vi "GUI_HTT_MultiCamDriveExpAndComp.vi"() -> ()   [LabVIEW 2020]
uses:
  Shared/GUI_Template/GUI_master/tcp_new_data_event.ctl
  Shared/GUI_Template/GUI_master/tcp new data cluster.ctl
  General GUIs/Device GUIs/GUI_Cameras/Controls/Crosshair type def.ctl
  <userlib>/_OpenG.lib/array/array.llb/Filter 1D Array with Scalar (String)__ogtk.vi
panel:
  out "image1 4":T1(plugin-control)
  out "image1 3":T1(plugin-control)
  out "image1 2":T1(plugin-control)
  out "image::5":T1(plugin-control) caption="HTT-MagCam-04"
  out "image::4":T1(plugin-control) caption="HTT-MagCam-04"
  out "image::3":T1(plugin-control) caption="HTT-MagCam-04"
  out "image::2":T1(plugin-control) caption="HTT-MagCam-04"
  out "image1":T1(plugin-control)
  out "String 4":string="x1\ny1\nx2\ny2"
  out "String 3":string="x1\ny1\nx2\ny2"
  out "String 2":string="x1\ny1\nx2\ny2"
  out "String":string="x1\ny1\nx2\ny2"
  in  "visibility":bool=TRUE
  out "appended array":string[](array[string]) caption="XH"
  out "appended array 6":string[](array[string]) caption="XH"
  out "appended array 8":string[](array[string]) caption="XH"
  out "appended array 4":string[](array[string]) caption="XH"
  in  "UDP error message":string
  out "tcp data event 2":T2
  out "error IO 2":errorcluster
  in  "Color Box":u32(colorbox)
  in  "TargetSize.Y::5":dbl=45.0 caption="y" min=2.0 max=3000.0 format="%#_6f"
  in  "TargetSize.X::5":dbl=47.0 caption="x" min=2.0 max=3000.0 format="%#_6f"
  in  "TargetSize.Y::4":dbl=45.0 caption="y" min=2.0 max=3000.0 format="%#_6f"
  in  "TargetSize.X::4":dbl=47.0 caption="x" min=2.0 max=3000.0 format="%#_6f"
  in  "TargetSize.Y::3":dbl=163.0 caption="y" min=2.0 max=3000.0 format="%#_6f"
  in  "TargetSize.X::3":dbl=152.0 caption="x" min=2.0 max=3000.0 format="%#_6f"
  in  "TargetSize.Y::2":dbl=74.0 caption="y" min=2.0 max=3000.0 format="%#_6f"
  in  "TargetSize.X::2":dbl=75.0 caption="x" min=2.0 max=3000.0 format="%#_6f"
  in  "active cams":string
  out "CCDs":string[](array[string])
  out "Cameras":T3
  in  "Target.Y::5":dbl=45.0 caption="y" min=0.0 max=2000.0 format="%#_6f"
  in  "Target.X::5":dbl=47.0 caption="x" min=0.0 max=2000.0 format="%#_6f"
  in  "Target.Y::4":dbl=45.0 caption="y" min=0.0 max=2000.0 format="%#_6f"
  in  "Target.X::4":dbl=47.0 caption="x" min=0.0 max=2000.0 format="%#_6f"
  in  "Target.Y::3":dbl=163.0 caption="y" min=0.0 max=2000.0 format="%#_6f"
  in  "Target.X::3":dbl=152.0 caption="x" min=0.0 max=2000.0 format="%#_6f"
  in  "Target.Y::2":dbl=74.0 caption="y" min=0.0 max=2000.0 format="%#_6f"
  in  "Target.X::2":dbl=75.0 caption="x" min=0.0 max=2000.0 format="%#_6f"
  out "error out":errorcluster
  in  "triggerdelay::5":dbl=0.001 caption="triggerdelay" min=0.0 max=1000000.0 format="%_4p"
  in  "triggerdelay::4":dbl=0.001 caption="triggerdelay" min=0.0 max=10000000.0 format="%_4p"
  in  "triggerdelay::3":dbl=0.001 caption="triggerdelay" min=0.0 max=1000000.0 format="%_4p"
  in  "triggerdelay::2":dbl=0.001 caption="triggerdelay" min=0.0 max=1000000.0 format="%_4p"
  in  "trigger::5":bool caption="Trigger"
  in  "centroidy::5":dbl=0.001 caption="centroid y" min=0.0 max=0.0 format="%_4f"
  in  "centroidx::5":dbl=0.001 caption="centroid x" min=0.0 max=0.0 format="%_4f"
  in  "exposure::5":dbl=0.001 caption="exposure" min=1.0 max=10000000.0 format="%_4p"
  in  "GUIdevice 5":string="BellaCam25_2_cpoint2"
  in  "trigger::4":bool caption="Trigger"
  in  "centroidy::4":dbl=0.001 caption="centroid y" min=0.0 max=0.0 format="%_4f"
  in  "centroidx::4":dbl=0.001 caption="centroid x" min=0.0 max=0.0 format="%_4f"
  in  "exposure::4":dbl=0.001 caption="exposure" min=0.0001 max=1.0 format="%_4p"
  in  "GUIdevice 4":string="BellaCam13_1_cpoint1"
  in  "trigger::3":bool caption="Trigger"
  in  "centroidy::3":dbl=0.001 caption="centroid y" min=0.0 max=0.0 format="%_4f"
  in  "centroidx::3":dbl=0.001 caption="centroid x" min=0.0 max=0.0 format="%_4f"
  in  "exposure::3":dbl=0.001 caption="exposure" min=1e-05 max=1.0 format="%_4p"
  in  "GUIdevice 3":string="BellaCam13_3_tpoint2"
  in  "trigger::2":bool caption="Trigger"
  in  "centroidy::2":dbl=0.001 caption="centroid y" min=0.0 max=0.0 format="%_4f"
  in  "centroidx::2":dbl=0.001 caption="centroid x" min=0.0 max=0.0 format="%_4f"
  in  "exposure::2":dbl=0.001 caption="exposure" min=1.0 max=10000000.0 format="%_4p"
  in  "GUIdevice 2":string="BellaCam25_1_tpoint1"
  out "tcp data event":T2
  in  "Refresh Button":bool caption="Update Crosshairs"
  in  "Select device":string(combo)="FrogHPD"
  in  "stop":bool
  in  "GUIdevice 1":string="HPD_CCD"
  # "XHair location"
  # "XHair location"
  # "XHair size"
  # "XHair size"
  # "XHair location"
  # "XHair size"
  # "XHair size"
  # "XHair location"
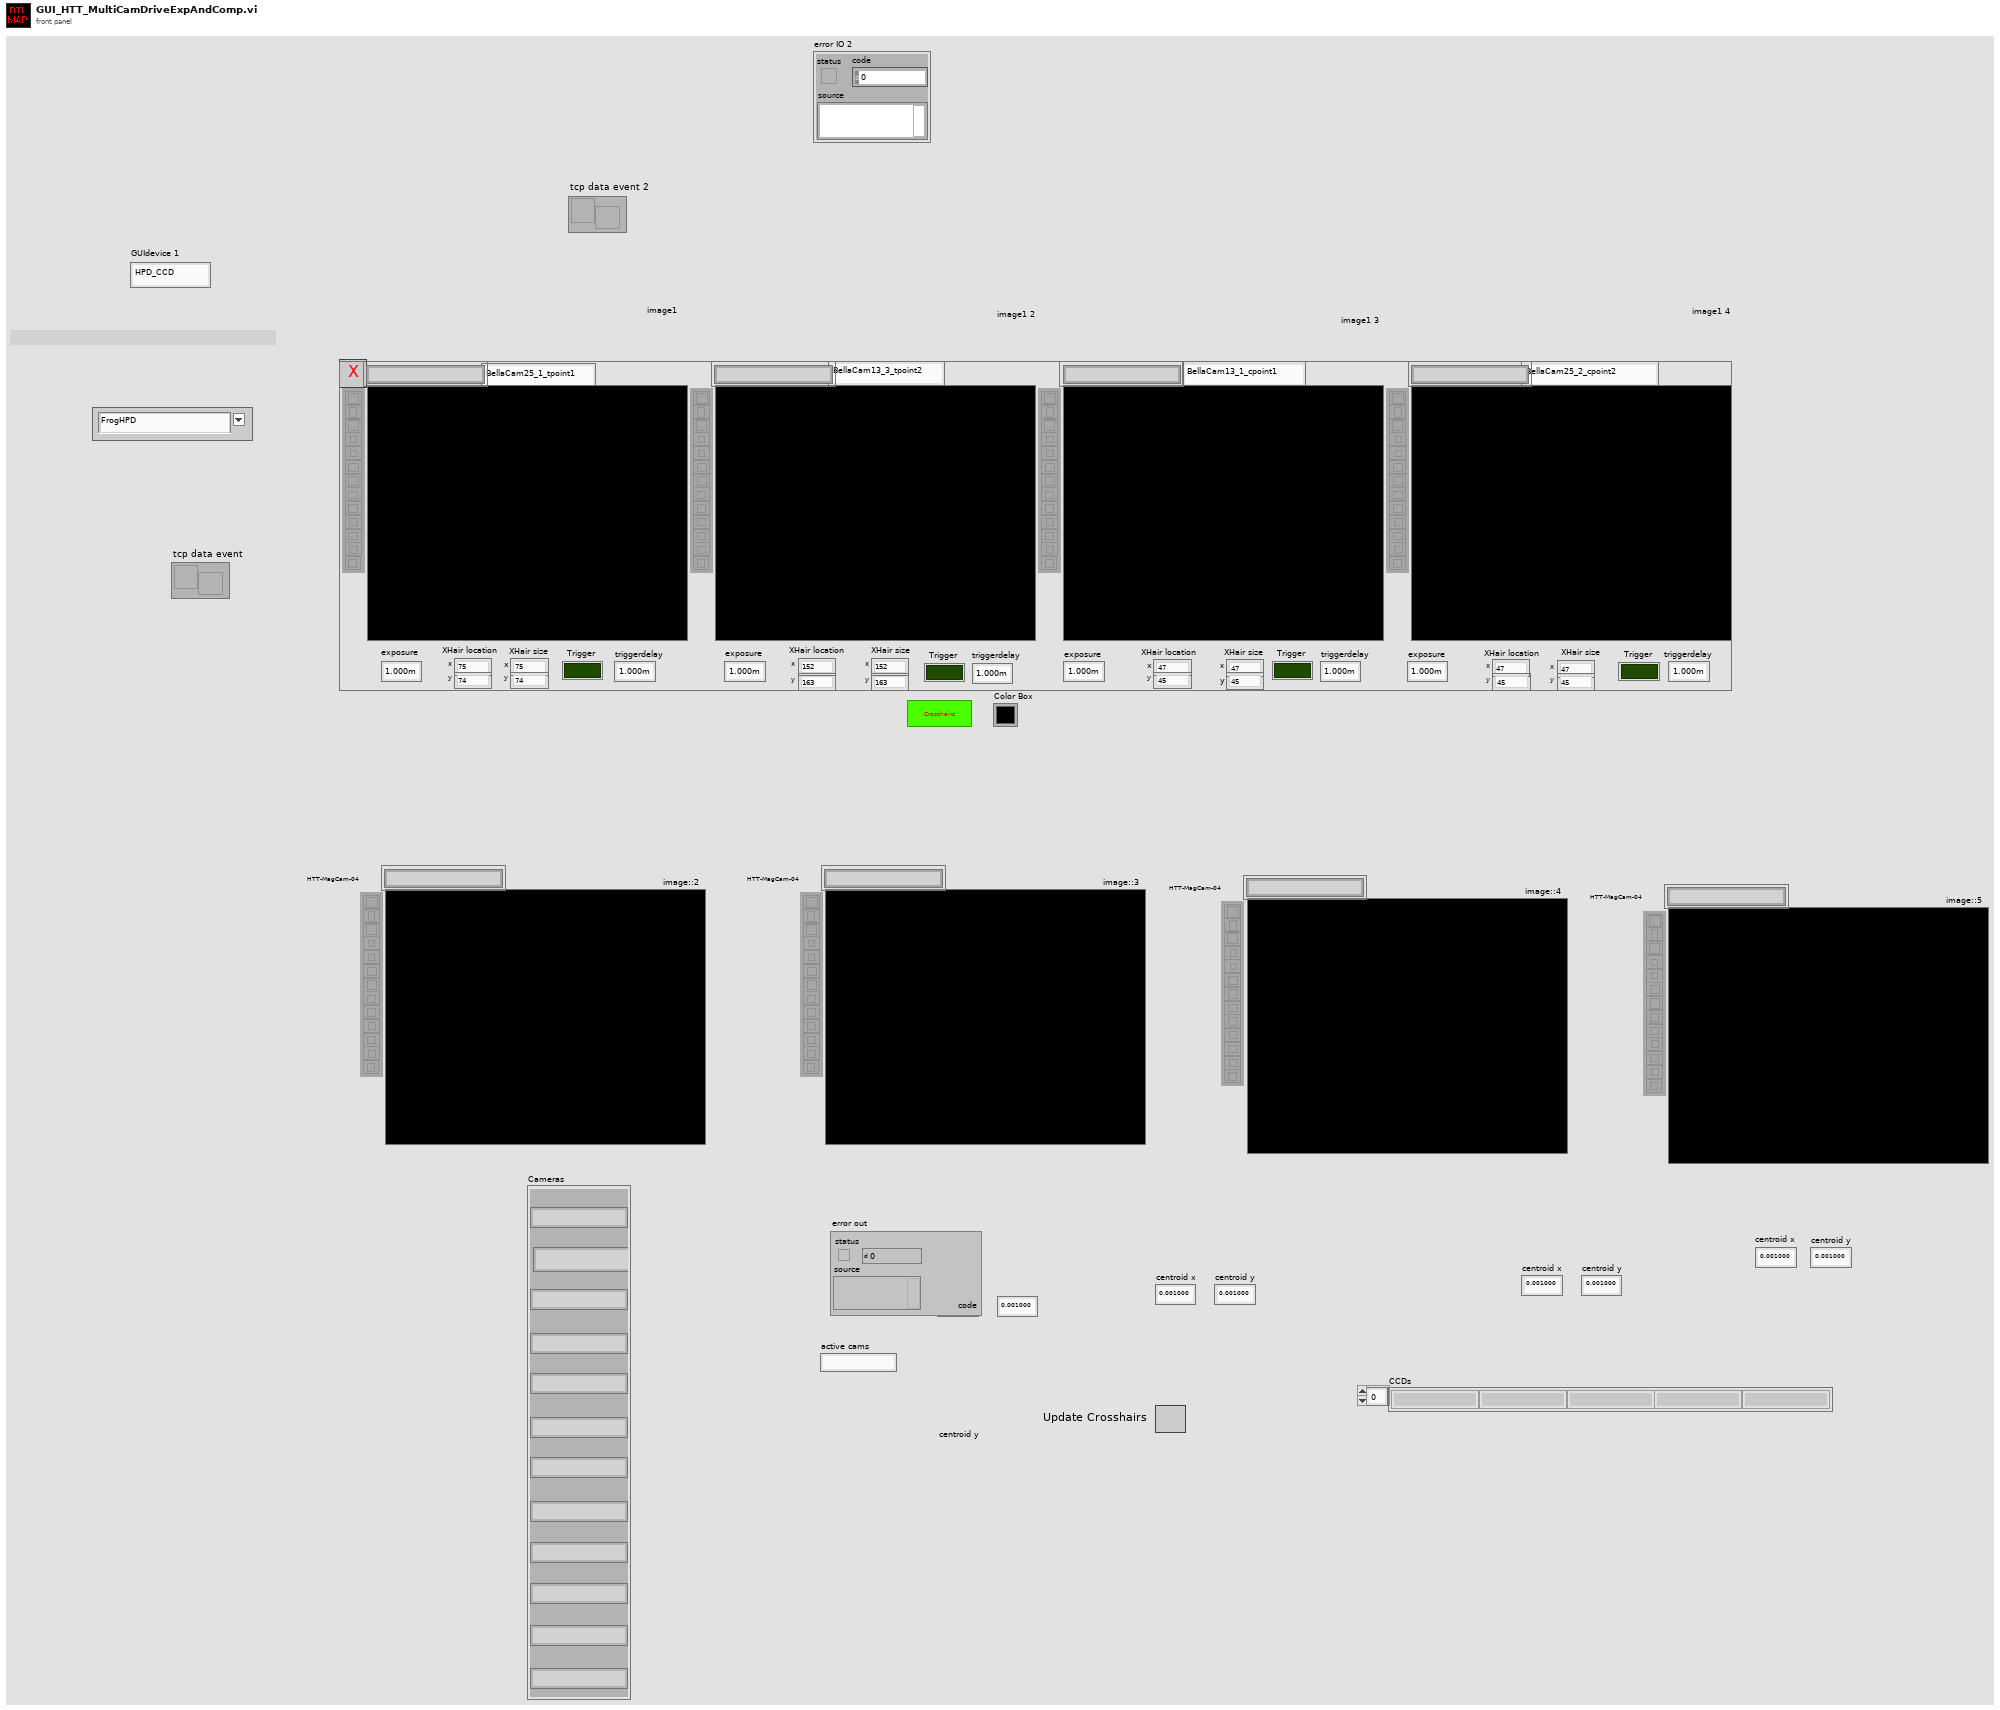
[diagram p1: front panel]
types:
  T1 = typedef "IMAQ Image.ctl" = refnum<image>
  T2 = typedef "tcp_new_data_event.ctl" = refnum<user-event>
  T3 = cluster{"[0]":string, "[1]":string, "[2]":string, "[3]":string, "[4]":string, "[5]":string, "[6]":string, "[7]":string, "[8]":string, "[8] 2":string, "[8] 3":string, "[8] 4":string}
  T4 = typedef "Image Type" = u32
  T5 = cluster{"Target.X::2":refnum<vi>, "Target.Y::2":refnum<vi>}
  T6 = cluster{"Target.X::3":refnum<vi>, "Target.Y::3":refnum<vi>}
  T7 = cluster{"Target.X::4":refnum<vi>, "Target.Y::4":refnum<vi>}
  T8 = cluster{"Target.X::5":refnum<vi>, "Target.Y::5":refnum<vi>}
  T9 = cluster{"TargetSize.X::2":refnum<vi>, "TargetSize.Y::2":refnum<vi>}
  T10 = cluster{"TargetSize.X::3":refnum<vi>, "TargetSize.Y::3":refnum<vi>}
  T11 = cluster{"TargetSize.X::4":refnum<vi>, "TargetSize.Y::4":refnum<vi>}
  T12 = cluster{"TargetSize.X::5":refnum<vi>, "TargetSize.Y::5":refnum<vi>}
  T13 = cluster{"Target.X::5":refnum<vi>, "Target.Y::5":refnum<vi>}[]
  T14 = cluster{"TargetSize.X::5":refnum<vi>, "TargetSize.Y::5":refnum<vi>}[]
  T15 = cluster{"[0]":string, "[1]":string, "[2]":string, "[3]":string, "[4]":string, "[5]":string, "[6]":string, "[7]":string, "[8]":string, "[9]":string, "[10]":string, "[11]":string}
  T16 = typedef "Crosshair type def.ctl" = cluster{"Draw":bool, "Target":cluster{"x":dbl, "y":dbl}, "Size":cluster{"x":dbl, "y":dbl}, "Angle":dbl, "Color":u32, "Thickness":u8, "CrosshairLabel":string}
  T17 = cluster{"Left":i32, "Top":i32, "Right":i32, "Bottom":i32}
  T18 = enum32{"invalid app kind", "Development System", "Run Time System", "Student Edition", "Embedded LabVIEW", "Evaluation", "Custom"}
  T19 = typedef "tcp new data cluster.ctl" = cluster{"EventEnum":enum16{"new data", "connection status update"}, "Device name":string}
  T20 = enum32{"Invalid", "Standard", "Closed", "Hidden", "Minimized", "Maximized"}
  T21 = cluster{"Core":cluster{"Current VI Reference":refnum<vi>, "Close Panel on Exit?":bool}, "Your Boolean data":bool, "active cams":string, "SuperGUI":cluster{"STOP queue":refnum<queue>, "SuperGUI ref":refnum<vi>}}
  T22 = cluster{"STOP queue":refnum<queue>, "SuperGUI ref":refnum<vi>}
  T23 = cluster{"Current VI Reference":refnum<vi>, "Close Panel on Exit?":bool}
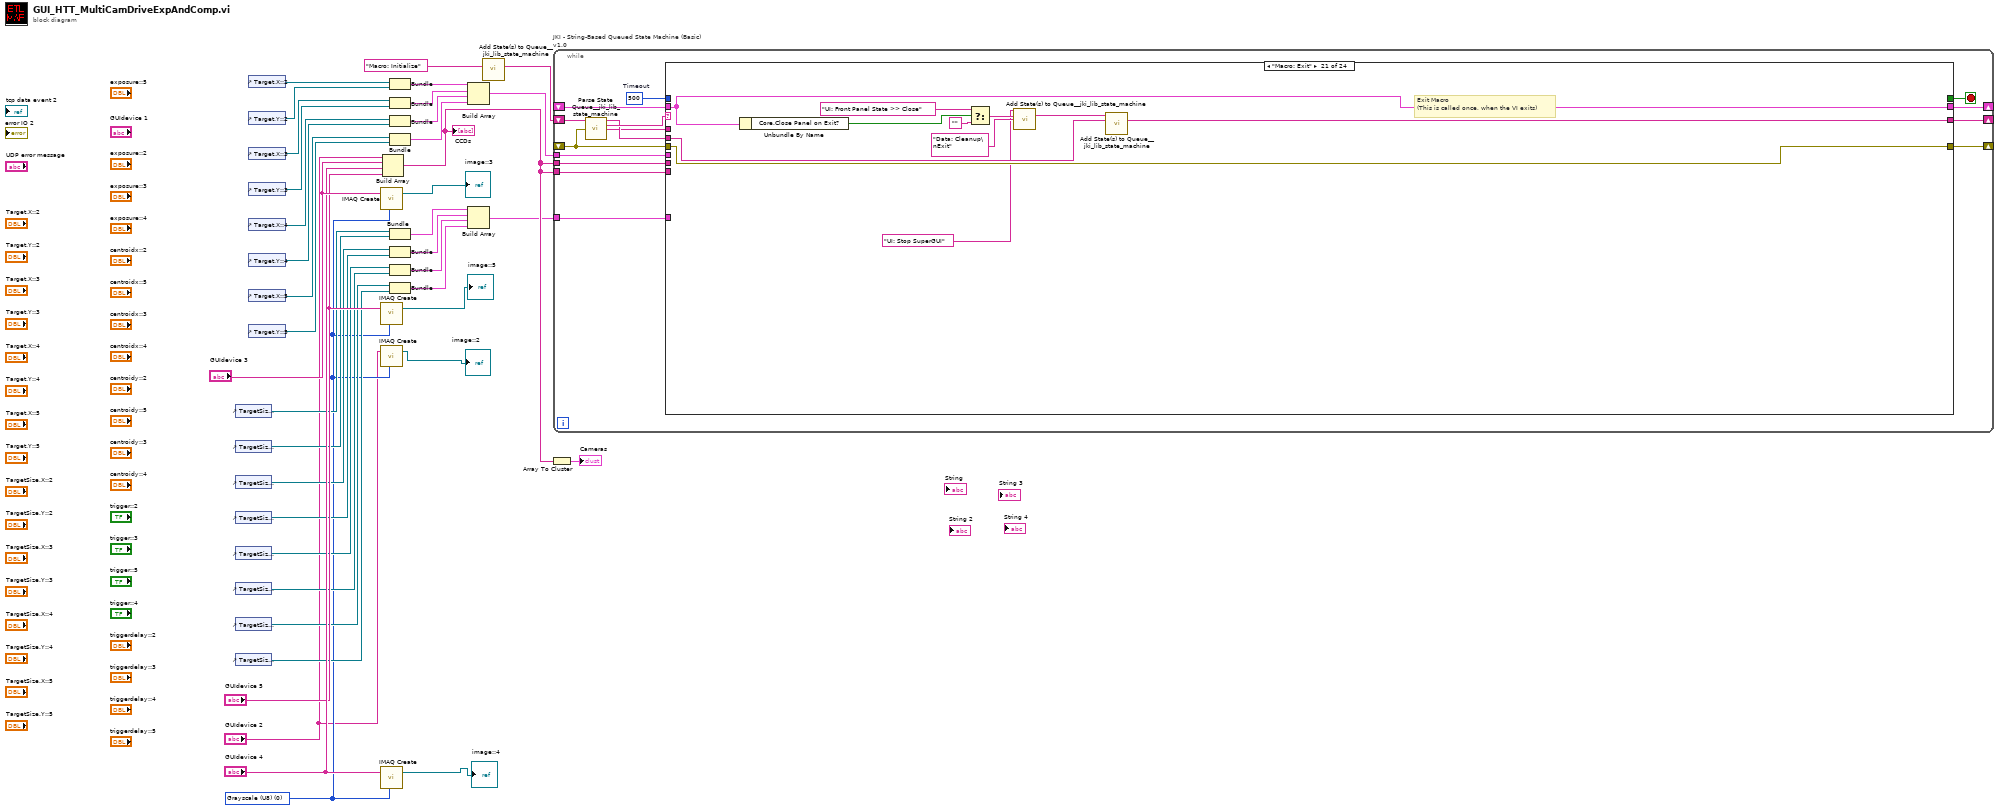
[diagram p0: block diagram]
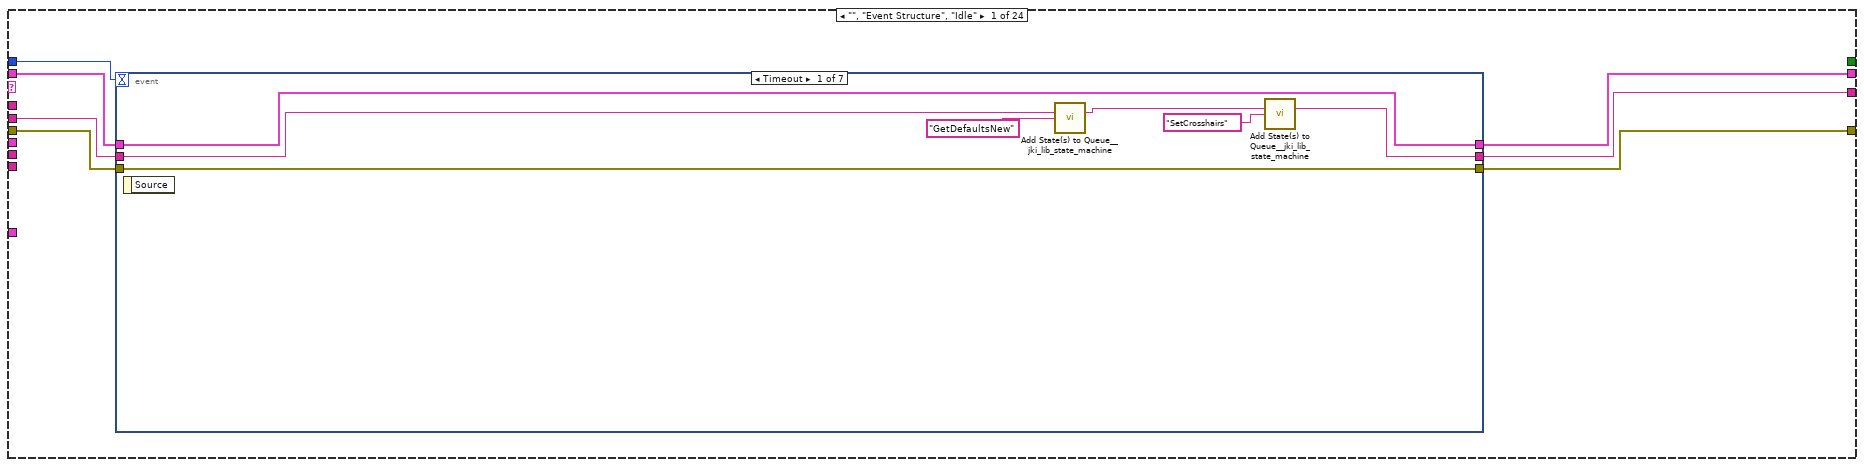
[diagram p2: hidden frame]
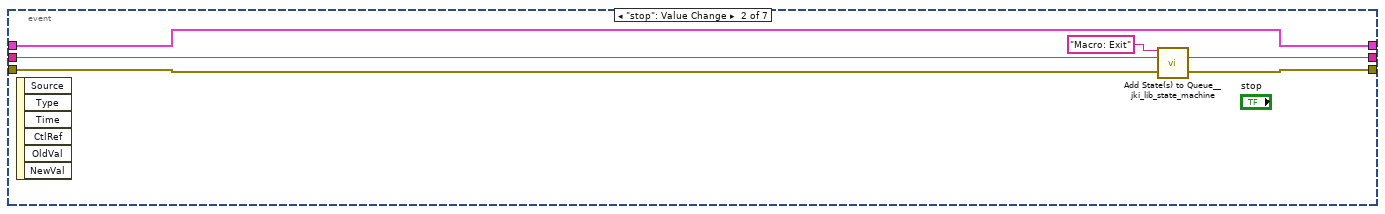
[diagram p3: hidden frame]
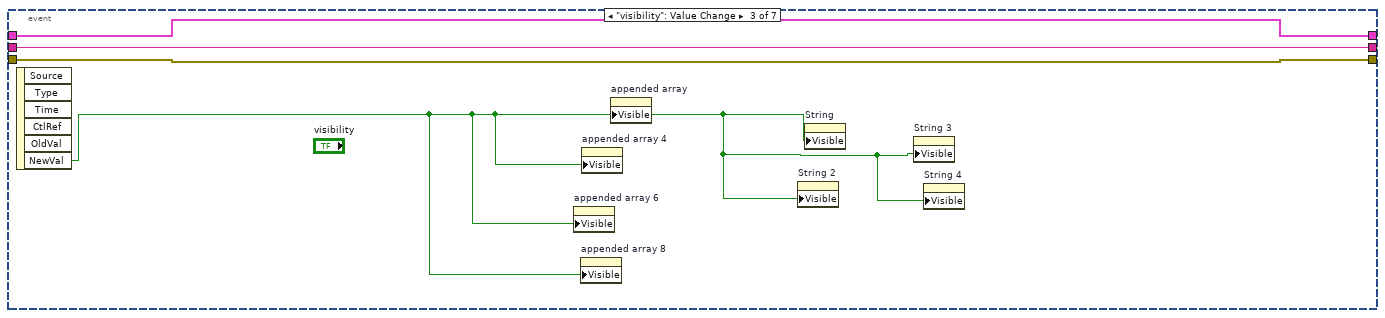
[diagram p4: hidden frame]
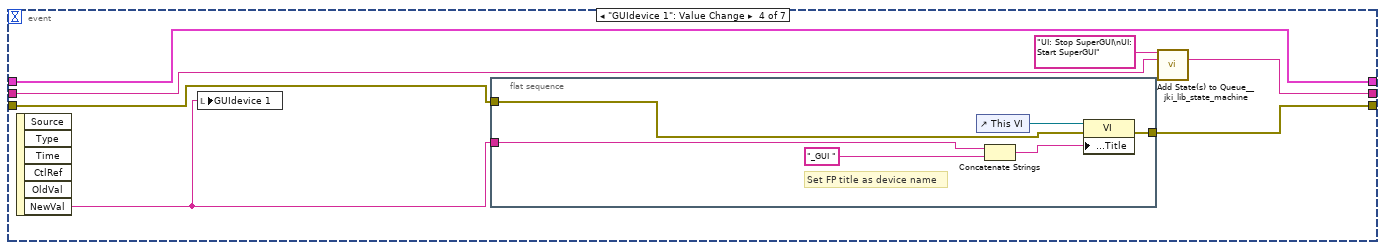
[diagram p5: hidden frame]
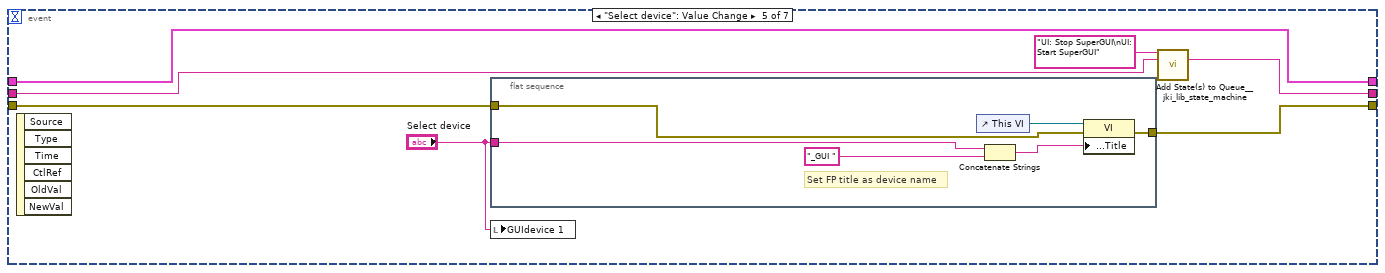
[diagram p6: hidden frame]
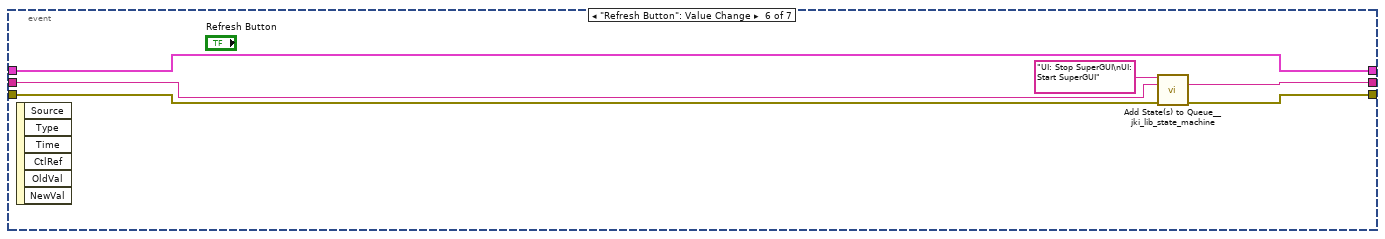
[diagram p7: hidden frame]
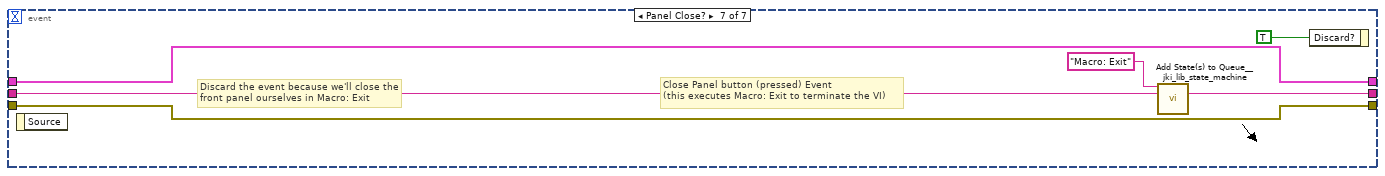
[diagram p8: hidden frame]
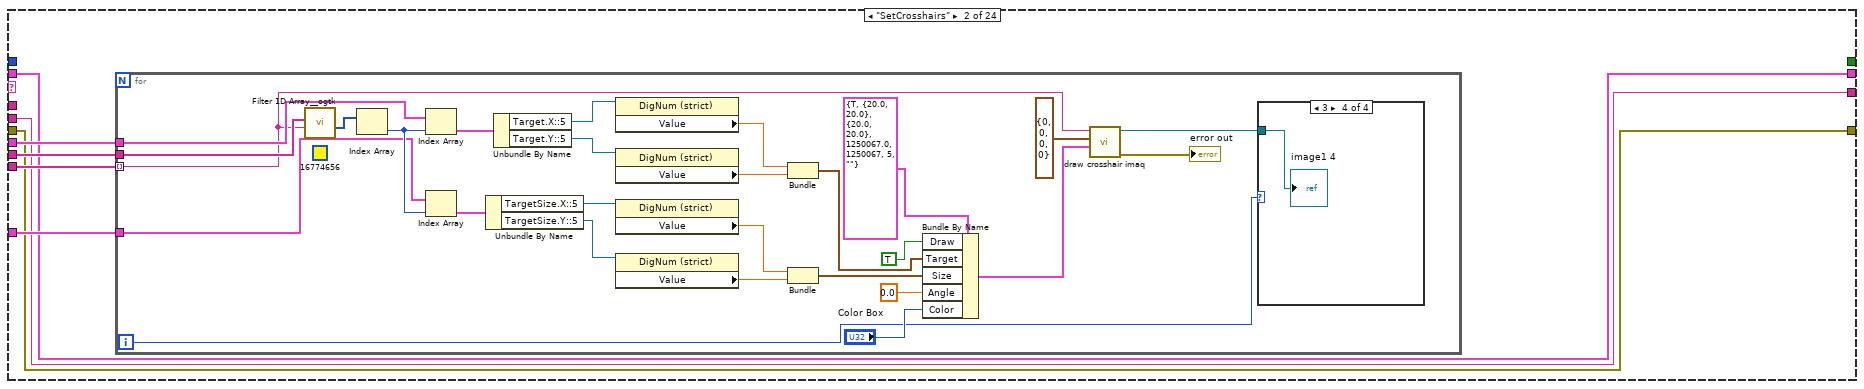
[diagram p9: hidden frame]
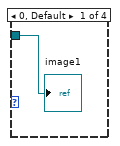
[diagram p10: hidden frame]
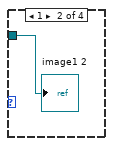
[diagram p11: hidden frame]
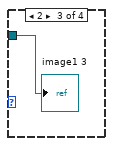
[diagram p12: hidden frame]
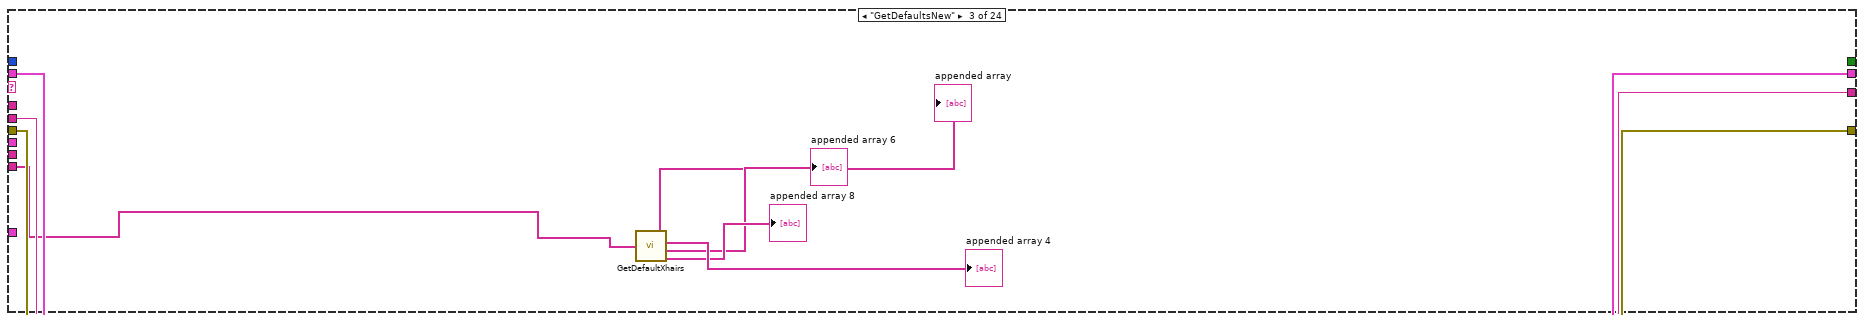
[diagram p13: hidden frame]
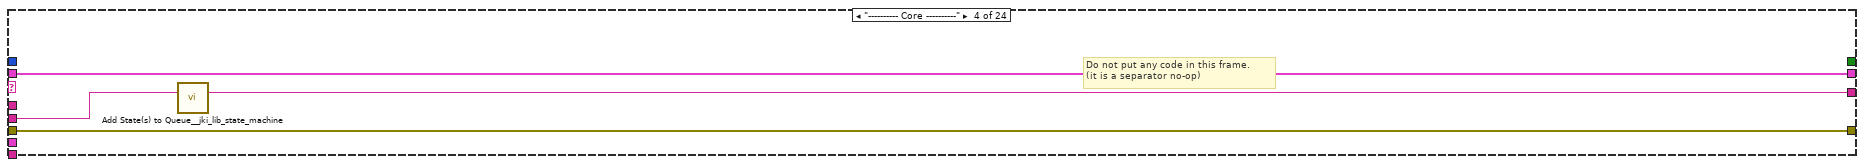
[diagram p14: hidden frame]
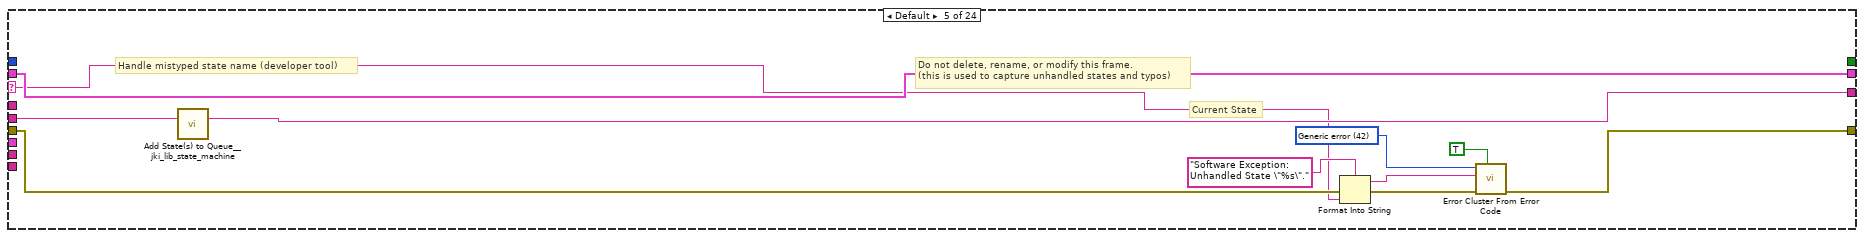
[diagram p15: hidden frame]
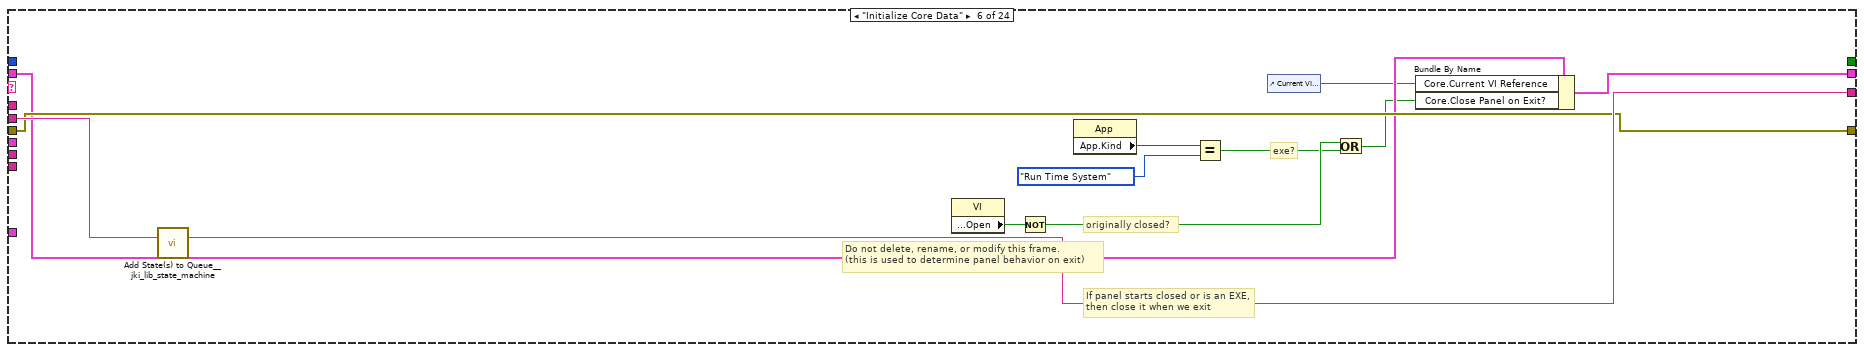
[diagram p16: hidden frame]
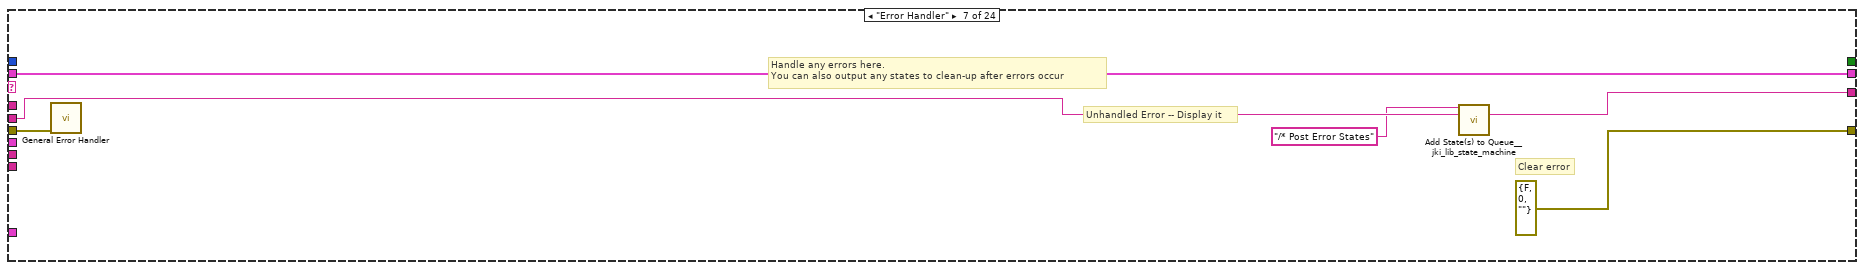
[diagram p17: hidden frame]
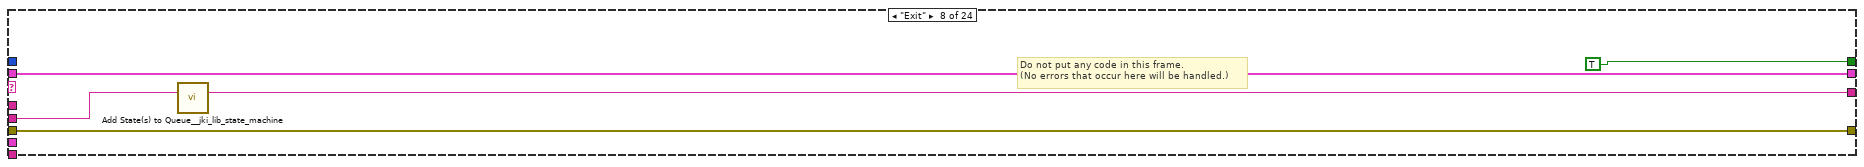
[diagram p18: hidden frame]
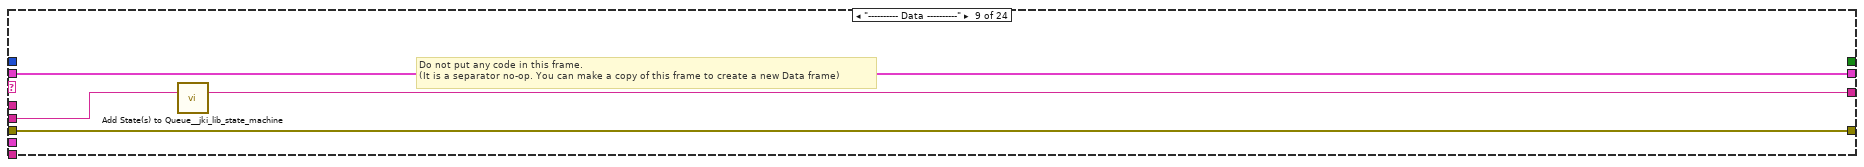
[diagram p19: hidden frame]
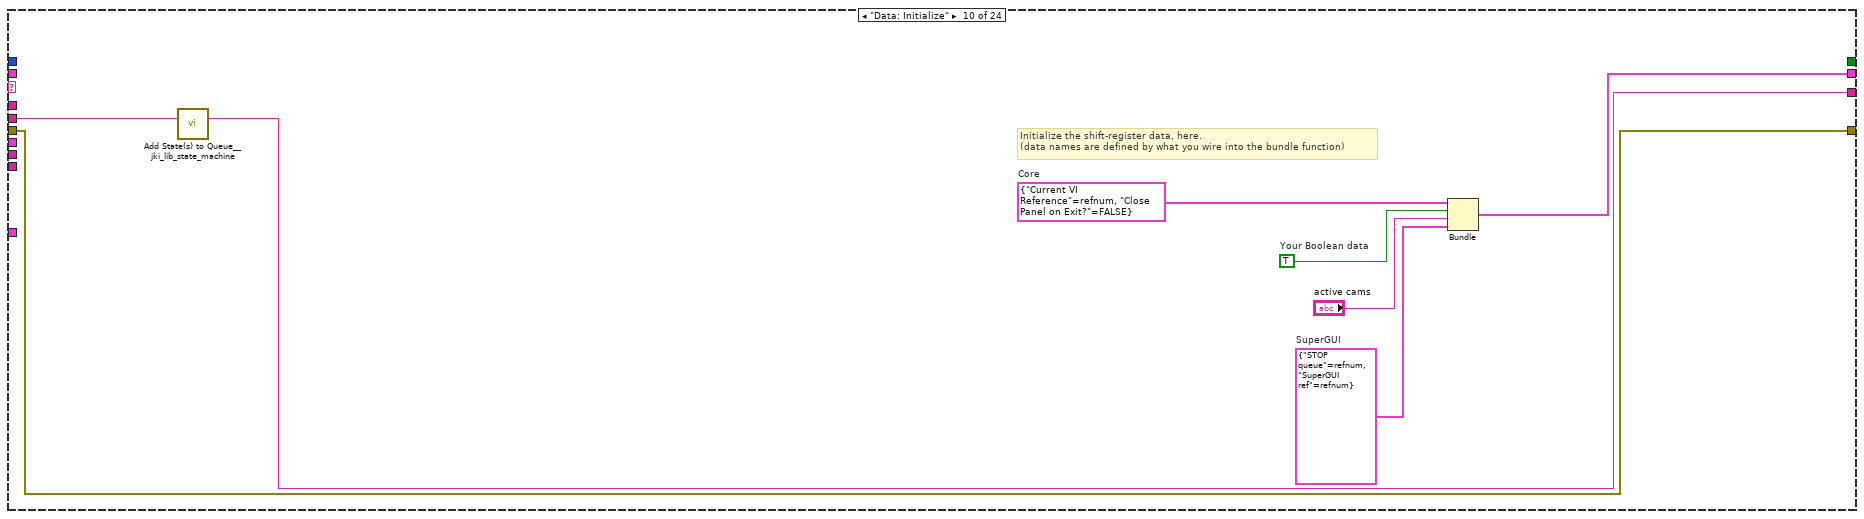
[diagram p20: hidden frame]
diagram:
  w6 = T4 0 items=["Grayscale (U8)", "Grayscale (I16)", "Grayscale (SGL)", "Complex (CSG)", "RGB (U32)", "HSL (U32)", "RGB (U64)", "Grayscale (U16)"] ("Image Type")
  n1 = control-ref of="TargetSize.X::2"() -> (w19:refnum<vi>)
  n2 = control-ref of="TargetSize.Y::2"() -> (w18:refnum<vi>)
  n3 = control-ref of="TargetSize.X::3"() -> (w17:refnum<vi>)
  n4 = control-ref of="TargetSize.Y::3"() -> (w16:refnum<vi>)
  n5 = control-ref of="TargetSize.X::4"() -> (w15:refnum<vi>)
  n6 = control-ref of="TargetSize.Y::4"() -> (w14:refnum<vi>)
  n7 = control-ref of="TargetSize.X::5"() -> (w13:refnum<vi>)
  n8 = control-ref of="TargetSize.Y::5"() -> (w12:refnum<vi>)
  n9 = control-ref of="Target.X::2"() -> (w37:refnum<vi>)
  n10 = control-ref of="Target.Y::2"() -> (w36:refnum<vi>)
  n11 = control-ref of="Target.X::3"() -> (w35:refnum<vi>)
  n12 = control-ref of="Target.Y::3"() -> (w34:refnum<vi>)
  n13 = control-ref of="Target.X::4"() -> (w33:refnum<vi>)
  n14 = control-ref of="Target.Y::4"() -> (w32:refnum<vi>)
  n15 = control-ref of="Target.X::5"() -> (w31:refnum<vi>)
  n16 = control-ref of="Target.Y::5"() -> (w30:refnum<vi>)
  n17 = call "IMAQ Create"("Image Name"="GUIdevice 3", "Image Type"=w6) -> ("New Image"=→"image::3":T1)  [unwired: 3 in, 1 out]
  n18 = call "IMAQ Create"("Image Name"="GUIdevice 5", "Image Type"=w6) -> ("New Image"=→"image::5":T1)  [unwired: 3 in, 1 out]
  n19 = call "IMAQ Create"("Image Name"="GUIdevice 2", "Image Type"=w6) -> ("New Image"=→"image::2":T1)  [unwired: 3 in, 1 out]
  n20 = call "IMAQ Create"("Image Name"="GUIdevice 4", "Image Type"=w6) -> ("New Image"=→"image::4":T1)  [unwired: 3 in, 1 out]
  n21 = Build Array("GUIdevice 2", "GUIdevice 3", "GUIdevice 4", "GUIdevice 5") -> (w20:string[])
  "CCDs" <- w20
  n22 = Bundle("Target.X::2"=w37, "Target.Y::2"=w36) -> (w29:T5)  [unwired: 1 in]
  n23 = Bundle("Target.X::3"=w35, "Target.Y::3"=w34) -> (w28:T6)  [unwired: 1 in]
  n24 = Bundle("Target.X::4"=w33, "Target.Y::4"=w32) -> (w26:T7)  [unwired: 1 in]
  n25 = Bundle("Target.X::5"=w31, "Target.Y::5"=w30) -> (w27:T8)  [unwired: 1 in]
  n26 = Bundle("TargetSize.X::2"=w19, "TargetSize.Y::2"=w18) -> (w11:T9)  [unwired: 1 in]
  n27 = Bundle("TargetSize.X::3"=w17, "TargetSize.Y::3"=w16) -> (w10:T10)  [unwired: 1 in]
  n28 = Bundle("TargetSize.X::4"=w15, "TargetSize.Y::4"=w14) -> (w8:T11)  [unwired: 1 in]
  n29 = Bundle("TargetSize.X::5"=w13, "TargetSize.Y::5"=w12) -> (w9:T12)  [unwired: 1 in]
  n30 = Build Array(w29, w28, w26, w27) -> (w25:T13)
  n31 = Build Array(w11, w10, w8, w9) -> (w7:T14)
  n32 = call <vilib>:"Add State(s) to Queue__jki_lib_state_machine.vi"("State(s) in (\"\")"="Macro: Initialize") -> ("States Out"=w39:string)  [unwired: 14 in]
  n33 = Array To Cluster(array=w20) -> (cluster=→"Cameras":T15)
  n34 = while "JKI - String-Based Queued State Machine (Basic) v1.0" {
    shift-right: [w47] -> _
    shift-left: _ -> [w44]
    shift-right: [w50] -> _
    shift-left: _ -> [w45]
    shift-right: [w49] -> _
    shift-left: w39 -> [w51]
    tunnel: w25 -> [w41]
    tunnel: w20 -> [w42]
    tunnel: w20 -> [w43]
    tunnel: w7 -> [w40]
    stop <- w48 stop-if-true
    w46 = 500  # Timeout
    n35 = call <vilib>:"Parse State Queue__jki_lib_state_machine.vi"("State Queue"=w51, "Error In (no error)"=w45) -> ("Remaining States"=w53:string, "Current State"=w54:string, "Arguments"=w52:string)  [unwired: 11 in]
    n36 = case shown="\"Macro: Exit\"" w54 {
      selector: w54 -> [_ _ _ _ w165 _ _ _ _ _ _ _ _ _ _ _ _ _ _ _ _ _ _ _]
      tunnel: w53 -> [w61 w116 w159 w164 w169 w187 w193 w198 w202 w210 w216 w220 w227 w235 w270 w278 w284 w295 w321 w326 w337 w341 w345 w349]
      tunnel: w52 -> [_ _ _ _ _ _ _ _ _ _ _ _ _ _ _ _ w279 w289 _ _ _ _ _ _]
      tunnel: w44 -> [w59 w117 w160 w161 w167 w178 w190 w196 w199 _ w211 w217 w225 w233 w261 w273 w282 w291 w318 w323 w334 w338 w342 w346]
      tunnel: [w58 w115 w158 w162 w171 w184 errorcluster {"status"=FALSE, "code"=0, "source"=""} ("error out") w195 w200 w207 w212 w218 w223 w230 w254 w271 w280 w292 w319 w324 w335 w339 w343 w347] -> w50
      tunnel: w45 -> [w57 w115 w158 w162 w170 w184 w189 w195 w200 w207 w213 w218 w224 w231 w255 w272 w281 w293 w319 w324 w335 w339 w343 w347]
      tunnel: [w60 w116 w159 w163 w168 w186 w192 w197 w201 w209 w215 w219 w226 w234 w269 w277 w283 w294 w320 w325 w336 w340 w344 w348] -> w49
      tunnel: [_ _ _ _ _ _ _ TRUE _ _ _ _ _ _ _ _ _ _ _ _ _ _ _ _] -> w48
      tunnel: [w56 w117 w160 w161 w167 w185 w190 w196 w199 w208 w211 w217 w225 w233 w260 w273 w282 w291 w318 w323 w334 w338 w342 w346] -> w47
      tunnel: w46 -> [w55 _ _ _ _ _ _ _ _ _ _ _ _ _ _ _ _ _ _ _ _ _ _ _]
      tunnel: w43 -> [_ w119 w157 _ _ _ _ _ _ _ _ _ _ _ _ _ _ _ _ _ _ _ _ _]
      tunnel: w42 -> [_ w120 _ _ _ _ _ _ _ _ _ _ _ _ _ _ _ _ _ _ _ _ _ _]
      tunnel: w41 -> [_ w121 _ _ _ _ _ _ _ _ _ _ _ _ _ _ _ _ _ _ _ _ _ _]
      tunnel: w40 -> [_ w118 _ _ _ _ _ _ _ _ _ _ _ _ _ _ _ _ _ _ _ _ _ _]
      frame "", "Event Structure", "Idle" {
        n37 = event shown="[0] Timeout" {
          selector: _ -> [_ _ _ _ _ _ _]
          dyn-events: _ -> [_ _ _ _ _ _ _]
          timeout: w55 -> [_ _ _ _ _ _ _]
          tunnel: w61 -> [w64 w71 w75 w81 w93 w106 w114]
          tunnel: [w68 w70 w75 w80 w92 w105 w113] -> w60
          tunnel: w59 -> [w66 w73 w77 w84 w97 w108 w111]
          tunnel: [w67 w72 w76 w82 w95 w107 w112] -> w58
          tunnel: w57 -> [w67 w72 w76 w83 w96 w107 w112]
          tunnel: [w66 w73 w77 w84 w97 w108 w111] -> w56
          event Timeout {
            n38 = event-data() -> ()  [unwired: 1 in, 1 out]
            n39 = call <vilib>:"Add State(s) to Queue__jki_lib_state_machine.vi"("State(s) in (\"\")"=w64, "State(s) at Back (\"\")"="GetDefaultsNew") -> ("States Out"=w62:string)  [unwired: 13 in]
            n40 = call <vilib>:"Add State(s) to Queue__jki_lib_state_machine.vi"("State(s) in (\"\")"=w62, "State(s) at Back (\"\")"="SetCrosshairs") -> ("States Out"=w68:string)  [unwired: 13 in]
          }
          event "stop": Value Change {
            n41 = event-data() -> ()  [unwired: 1 in, 6 out]
            n42 = call <vilib>:"Add State(s) to Queue__jki_lib_state_machine.vi"("State(s) in Front (\"\")"="Macro: Exit", "State(s) in (\"\")"=w71) -> ("States Out"=w70:string)  [unwired: 13 in]
          }
          event "visibility": Value Change {
            n43 = event-data() -> ("NewVal"=w74:bool)  [unwired: 1 in, 5 out]
            n44 = property on="appended array 6" class="Arr (strict)"("Visible"=w74) -> ()  [unwired: 2 in, 2 out]
            n45 = property on="appended array 8" class="Arr (strict)"("Visible"=w74) -> ()  [unwired: 2 in, 2 out]
            n46 = property on="appended array 4" class="Arr (strict)"("Visible"=w74) -> ()  [unwired: 2 in, 2 out]
            n47 = property on="appended array" class="Arr (strict)"("Visible"=w74) -> ()  [unwired: 2 in, 2 out]
            n48 = property on="String 2" class="Str"("Visible"=w74) -> ()  [unwired: 2 in, 2 out]
            n49 = property on="String" class="Str"("Visible"=w74) -> ()  [unwired: 2 in, 2 out]
            n50 = property on="String 3" class="Str"("Visible"=w74) -> ()  [unwired: 2 in, 2 out]
            n51 = property on="String 4" class="Str"("Visible"=w74) -> ()  [unwired: 2 in, 2 out]
          }
          event "GUIdevice 1": Value Change {
            n52 = event-data() -> ("NewVal"=w78:string)  [unwired: 1 in, 5 out]
            n53 = local write "GUIdevice 1"(w78) -> ()
            n54 = flat-sequence {
              tunnel: [w87] -> w82
              tunnel: w83 -> [w86]
              tunnel: w78 -> [w85]
              frame #0 {
                # "Set FP title as device name"
                n55 = control-ref of="This VI"() -> (w90:refnum<vi>)
                n56 = Concatenate Strings(w85, "_GUI ") -> (w89:string)
                n57 = property class="VI"(reference=w90, error in=w86, "Front Panel.Title"=w89) -> (error out=w87:errorcluster)  [unwired: 1 out]
              }
            }
            n58 = call <vilib>:"Add State(s) to Queue__jki_lib_state_machine.vi"("State(s) in Front (\"\")"="UI: Stop SuperGUI\nUI: Start SuperGUI", "State(s) in (\"\")"=w81) -> ("States Out"=w80:string)  [unwired: 13 in]
          }
          event "Select device": Value Change {
            n59 = event-data() -> ()  [unwired: 1 in, 6 out]
            n60 = flat-sequence {
              tunnel: [w100] -> w95
              tunnel: w96 -> [w99]
              tunnel: "Select device" -> [w98]
              frame #0 {
                # "Set FP title as device name"
                n61 = control-ref of="This VI"() -> (w103:refnum<vi>)
                n62 = Concatenate Strings(w98, "_GUI ") -> (w102:string)
                n63 = property class="VI"(reference=w103, error in=w99, "Front Panel.Title"=w102) -> (error out=w100:errorcluster)  [unwired: 1 out]
              }
            }
            n64 = local write "GUIdevice 1"("Select device") -> ()
            n65 = call <vilib>:"Add State(s) to Queue__jki_lib_state_machine.vi"("State(s) in Front (\"\")"="UI: Stop SuperGUI\nUI: Start SuperGUI", "State(s) in (\"\")"=w93) -> ("States Out"=w92:string)  [unwired: 13 in]
          }
          event "Refresh Button": Value Change {
            n66 = event-data() -> ()  [unwired: 1 in, 6 out]
            n67 = call <vilib>:"Add State(s) to Queue__jki_lib_state_machine.vi"("State(s) in Front (\"\")"="UI: Stop SuperGUI\nUI: Start SuperGUI", "State(s) in (\"\")"=w106) -> ("States Out"=w105:string)  [unwired: 13 in]
          }
          event Panel Close? {
            # "Discard the event because we'll close the front panel ourselves in Macro: Exit"
            # "Close Panel button (pressed) Event\n(this executes Macro: Exit to terminate the VI)"
            n68 = event-data() -> ()  [unwired: 1 in, 1 out]
            n69 = call <vilib>:"Add State(s) to Queue__jki_lib_state_machine.vi"("State(s) in Front (\"\")"="Macro: Exit", "State(s) in (\"\")"=w114) -> ("States Out"=w113:string)  [unwired: 13 in]
            n70 = event-data("Discard?"=TRUE) -> ()  [unwired: 1 in, 1 out]
          }
        }
      }
      frame "SetCrosshairs" {
        n71 = for {
          tunnel: w120 -> [w127]
          tunnel: w121 -> [w126]
          tunnel: w118 -> [w125]
          tunnel: w119 -> [w124] mode=indexing
          i -> [w123]
          (unwired) u32 16774656 ("Color")
          n72 = call-poly <userlib>:"Filter 1D Array__ogtk.vi"("items to filter"=w124, "array"=w127) -> ("filtered item indices"=w131:i32[])  [unwired: 4 in, 1 out]
          n73 = Index Array(array=w131) -> (element=w134:i32)  [unwired: 1 in]
          n74 = Index Array(array=w126, index=w134) -> (element=w132:T8)
          n75 = Index Array(array=w125, index=w134) -> (element=w135:T12)
          n76 = Unbundle By Name(w135) -> ("TargetSize.X::5"=w136:refnum<vi>, "TargetSize.Y::5"=w137:refnum<vi>)
          n77 = Unbundle By Name(w132) -> ("Target.X::5"=w129:refnum<vi>, "Target.Y::5"=w130:refnum<vi>)
          n78 = property class="DigNum (strict)"(reference=w129) -> ("Value"=w143:dbl)  [unwired: 1 in, 2 out]
          n79 = property class="DigNum (strict)"(reference=w130) -> ("Value"=w144:dbl)  [unwired: 1 in, 2 out]
          n80 = property class="DigNum (strict)"(reference=w136) -> ("Value"=w138:dbl)  [unwired: 1 in, 2 out]
          n81 = property class="DigNum (strict)"(reference=w137) -> ("Value"=w139:dbl)  [unwired: 1 in, 2 out]
          n82 = Bundle("Value"=w143, "Value"=w144) -> (w145:cluster{"Value":dbl, "Value":dbl})  [unwired: 1 in]
          n83 = Bundle("Value"=w138, "Value"=w139) -> (w146:cluster{"Value":dbl, "Value":dbl})  [unwired: 1 in]
          n84 = Bundle By Name(cluster=T16 {"Draw"=TRUE, "Target"={"x"=20.0, "y"=20.0}, "Size"={"x"=20.0, "y"=20.0}, "Angle"=1250067.0, "Color"=1250067, "Thickness"=5, "CrosshairLabel"=""} ("Crosshair"), "Draw"=TRUE, "Target"=w145, "Size"=w146, "Angle"=0.0, "Color"="Color Box") -> (w141:T16)
          n85 = call "draw crosshair imaq.vi"("Crosshair"=w141, "Bounding Rectangle"=T17 {"Left"=0, "Top"=0, "Right"=0, "Bottom"=0}, "image in"=w124) -> ("error out"=→"error out":errorcluster, "image out"=w122:T1)  [unwired: 7 in]
          n86 = case shown="3" w123 {
            tunnel: w122 -> [w149 w150 w151 w152]
            frame 0, Default {
              "image1" <- w149
            }
            frame 1 {
              "image1 2" <- w150
            }
            frame 2 {
              "image1 3" <- w151
            }
            frame 3 {
              "image1 4" <- w152
            }
          }
        }
      }
      frame "GetDefaultsNew" {
        n87 = call "GetDefaultXhairs.vi"("appended array 2"=w157) -> ("appended array"=→"appended array":string[], "appended array 4"=→"appended array 4":string[], "appended array 6"=→"appended array 6":string[], "appended array 8"=→"appended array 8":string[])
      }
      frame "---------- Core ----------" {
        # "Do not put any code in this frame.\n(it is a separator no-op)"
        n88 = call <vilib>:"Add State(s) to Queue__jki_lib_state_machine.vi"("State(s) in (\"\")"=w164) -> ("States Out"=w163:string)  [unwired: 14 in]
      }
      frame Default {
        w174 = 42 items=["No error", "Argument error", "Memory is full", "Out of zone", "End of file", "File already open", "Generic file I/O error", "File not found", "File permission error", "Disk is full", "Duplicate path", "Too many files open", "System feature not enabled", "Resource file not found", "Cannot add resource", "Resource not found", "Image not found", "Image memory error", "Pen does not exist", "Config type invalid", "Config token not found", "Config parse error", "Config memory error", "Bad external code format", "Bad external code offset", "External code not present", "Null window", "Destroy window error", "Null menu", "Print aborted", "Bad print record", "Print driver error", "Windows error during printing", "Memory error during printing", "Print dialog error", "Generic print error", "Invalid device refnum", "Device not found", "Device parameter error", "Device unit error", "Cannot open device", "Device call aborted", "Generic error", "Cancelled by user", "Object ID too low", "Object ID too high", "Object not in heap", "Unknown heap", "Unknown object (invalid DefProc)", "Unknown object (DefProc not in table)", "Message out of range", "Invalid (null) method", "Unknown message", "Manager call not supported", "Bad address", "Network operation in progress", "Network operation timed out", "Connection is busy", "Network attribute not supported", "Network error", "Address in use", "System out of memory", "Connection aborted", "Connection refused", "Not connected", "Already connected", "Connection closed", "Initialization error (interapplication manager)", "Bad occurrence", "Wait on unbound occurrence handler", "Occurrence queue overflow", "Datalog type conflict", "Unused", "Unrecognized type (interapplication manager)", "Memory corrupt", "Failed to make temporary DLL", "Old CIN version", "Drag socket not found", "Failed to load drop-object", "Failed to register OLE object", "Failed to release OLE object", "Format specifier type mismatch", "Unknown format specifier", "Too few format specifiers", "Too many format specifiers", "Scan failed", "Newer CIN version", "Error converting to variant", "Runtime menu error", "Password tampered", "Variant attribute not found", "Incompatible variant data type", "Event data is not available", "Event Store is not present", "Occurrence is not found", "Event Queue is not created", "Event info is not available", "Refnum passed is NULL", "Error retrieving Class GUID", "Error retrieving CoClass GUID", "Error retrieving TypeLib GUID.", "Bad built application magic bytes.", "Specific driver is different from the specific driver associated with the Logical Name.", "There is no session opened to the class driver.", "Max Error", "MAX - Error with config objects", "MAX - Error loading configuration", "MAX - Group not supported"]
        # "Current State"
        # "Do not delete, rename, or modify this frame.\n(this is used to capture unhandled states and typos)"
        # "Handle mistyped state name (developer tool)"
        n89 = call <vilib>:"Add State(s) to Queue__jki_lib_state_machine.vi"("State(s) in (\"\")"=w169) -> ("States Out"=w168:string)  [unwired: 14 in]
        n90 = Format Into String(format string="Software Exception: Unhandled State \"%s\"." ("message"), error in=w170, w165) -> (resulting string=w173:string, error out=w172:errorcluster)  [unwired: 1 in]
        n91 = call <vilib>:"Error Cluster From Error Code.vi"("show call chain? (False)"=TRUE, "error in (no error)"=w172, "error message (\"\")"=w173, "error code (0)"=w174) -> ("error out"=w171:errorcluster)  [unwired: 5 in]
      }
      frame "Initialize Core Data" {
        # "Do not delete, rename, or modify this frame.\n(this is used to determine panel behavior on exit)"
        # "originally closed?"
        # "exe?"
        # "If panel starts closed or is an EXE, then close it when we exit"
        n92 = call <vilib>:"Add State(s) to Queue__jki_lib_state_machine.vi"("State(s) in (\"\")"=w187) -> ("States Out"=w186:string)  [unwired: 14 in]
        n93 = property class="VI"() -> ("Front Panel.Open"=w183:bool)  [unwired: 2 in, 2 out]
        n94 = Not(x=w183) -> (.not. x?=w180:bool)
        n95 = property class="App"() -> ("App.Kind"=w182:T18)  [unwired: 2 in, 2 out]
        n96 = Equal?(x=w182, y=T18."Run Time System" ("Application:Kind")) -> (x = y?=w179:bool)
        n97 = control-ref of="Current VI Reference"() -> (w176:refnum<vi>)
        n98 = Or(x=w180, y=w179) -> (x .or. y?=w177:bool)
        n99 = Bundle By Name(cluster=w178, "Core.Current VI Reference"=w176, "Core.Close Panel on Exit?"=w177) -> (w185:T21)
      }
      frame "Error Handler" {
        # "Unhandled Error -- Display it"
        # "Handle any errors here.\nYou can also output any states to clean-up after errors occur"
        # "Clear error"
        n100 = call <vilib>:"General Error Handler.vi"("error in (no error)"=w189) -> ()  [unwired: 10 in, 5 out]
        n101 = call <vilib>:"Add State(s) to Queue__jki_lib_state_machine.vi"("State(s) in Front (\"\")"="/* Post Error States", "State(s) in (\"\")"=w193) -> ("States Out"=w192:string)  [unwired: 13 in]
      }
      frame "Exit" {
        # "Do not put any code in this frame.\n(No errors that occur here will be handled.)"
        n102 = call <vilib>:"Add State(s) to Queue__jki_lib_state_machine.vi"("State(s) in (\"\")"=w198) -> ("States Out"=w197:string)  [unwired: 14 in]
      }
      frame "---------- Data ----------" {
        # "Do not put any code in this frame.\n(It is a separator no-op. You can make a copy of this frame to create a new Data frame)"
        n103 = call <vilib>:"Add State(s) to Queue__jki_lib_state_machine.vi"("State(s) in (\"\")"=w202) -> ("States Out"=w201:string)  [unwired: 14 in]
      }
      frame "Data: Initialize" {
        w203 = T22 {"STOP queue"=refnum, "SuperGUI ref"=refnum}  # SuperGUI
        w204 = T23 {"Current VI Reference"=refnum, "Close Panel on Exit?"=FALSE}  # Core
        w206 = TRUE  # Your Boolean data
        # "Initialize the shift-register data, here.\n(data names are defined by what you wire into the bundle function)"
        n104 = call <vilib>:"Add State(s) to Queue__jki_lib_state_machine.vi"("State(s) in (\"\")"=w210) -> ("States Out"=w209:string)  [unwired: 14 in]
        n105 = Bundle("Core"=w204, "Your Boolean data"=w206, "active cams"="active cams", "SuperGUI"=w203) -> (w208:T21)  [unwired: 1 in]
      }
      frame "Data: Cleanup" {
        # "Cleanup any data and references, here.\n(this is called automatically, by the Macro: Exit)"
        n106 = Unbundle By Name(w211) -> ("Core.Current VI Reference"=w214:refnum<vi>)
        n107 = call <vilib>:"Add State(s) to Queue__jki_lib_state_machine.vi"("State(s) in (\"\")"=w216) -> ("States Out"=w215:string)  [unwired: 14 in]
        n108 = Close Reference(reference=w214, error in (no error)=w213) -> (error out=w212:errorcluster)
      }
      frame "---------- UI ----------" {
        # "Do not put any code in this frame.\n(It is a separator no-op. You can make a copy of this frame to create a new UI frame)"
        n109 = call <vilib>:"Add State(s) to Queue__jki_lib_state_machine.vi"("State(s) in (\"\")"=w220) -> ("States Out"=w219:string)  [unwired: 14 in]
      }
      frame "UI: Initialize" {
        # "Initialize the User Interface, here.\n(this is called automatically, by the Macro: Init)"
        n110 = call <vilib>:"Add State(s) to Queue__jki_lib_state_machine.vi"("State(s) in (\"\")"=w227) -> ("States Out"=w226:string)  [unwired: 14 in]
        n111 = call <userlib>:"Fit VI window to Largest Dec__ogtk.vi"("error in (no error)"=w224) -> ("error out"=w223:errorcluster)  [unwired: 5 in, 1 out]
        n112 = for {
          tunnel: string[] ["Point Grey Camera", "Manta Camera", "Photometrics Cam", "Basler Camera"] -> [w229] mode=indexing
          tunnel: [w228] -> w221 mode=concatenating
          n113 = call "getDevices.vi"("Device Class"=w229) -> ("All Devices"=w228:string[])
        }
        n114 = property on="Select device" class="CmbBox"("Strings[]"=w221) -> ()  [unwired: 2 in, 2 out]
      }
      frame "UI: Get Device Name" {
        # "Initialize the User Interface, here.\n(this is called automatically, by the Macro: Init)"
        n115 = call <vilib>:"Add State(s) to Queue__jki_lib_state_machine.vi"("State(s) in (\"\")"=w235) -> ("States Out"=w234:string)  [unwired: 14 in]
        n116 = First Call?() -> (First Call?: T/F=w232:bool)
        n117 = case shown="True" w232 {
          tunnel: w231 -> [w236 w238]
          tunnel: [w236 w237] -> w230
          frame False {
          }
          frame True {
            n118 = disable-structure "Get Device name from control for vi mode\nand command line arg for exe" shown="RUN_TIME_ENGINE==True" {
              disable-tunnel: w238 -> [w239 w241]
              disable-tunnel: [w239 w240] -> w237
              frame condition #0 (active) {
              }
              frame condition #1 {
                n119 = control-ref of="This Application"() -> (w249:refnum<vi>)
                n120 = property class="App"(reference=w249) -> ("App.Args"=w248:string[])  [unwired: 1 in, 2 out]
                n121 = Index Array(array=w248, index #1=1 ("index")) -> (element #1=w242:string)  [unwired: 2 in, 2 out]
                n122 = Empty String/Path?(string/path=w242) -> (empty?=w246:bool)
                n123 = Concatenate Strings(w242, "_GUI ") -> (w244:string)
                n124 = case shown="False" w246 {
                  tunnel: w242 -> [w250 _]
                  frame False {
                    n125 = local write "GUIdevice 1"(w250) -> ()
                  }
                  frame True {
                  }
                }
                n126 = control-ref of="This VI"() -> (w245:refnum<vi>)
                n127 = property class="VI"(reference=w245, error in=w241, "Front Panel.Title"=w244) -> (error out=w240:errorcluster)  [unwired: 1 out]
              }
            }
          }
        }
      }
      frame "UI: Start SuperGUI" {
        # "create stop queue for supergui and its clones"
        # "x100 abort will be dependent on caller VI\nx80 abort will be independent of caller vi, this will abort vi when labview is closed."
        # "Start SuperGUI asynchronous way"
        n128 = vi-ref "GUI_Master_subvi_reentrant_queues.vi"() -> (w253:refnum<vi>)
        n129 = property class="VI"(reference=w253) -> ("Path"=w252:path)  [unwired: 1 in, 2 out]
        n130 = control-ref of="This Application"() -> (w259:refnum<vi>)
        n131 = Open VI Reference(type specifier VI Refnum (for type only)=refnum<vi> refnum, vi path=w252, options=256) -> (vi reference=w268:refnum<vi>, error out=w267:errorcluster)  [unwired: 3 in]
        n132 = Create User Event(user event datatype=T19 {"EventEnum"=enum."new data", "Device name"="Device name"} ("New Event"), error in=w255) -> (user event=w256:refnum<user-event>, error out=w262:errorcluster)
        "tcp data event" <- w256
        n133 = control-ref of="This VI"() -> (w258:refnum<vi>)
        n134 = register-events(w256) -> ()  [unwired: 2 in, 2 out]
        n135 = call "supergui create stop queue.vi"() -> ("STOP Queue out"=w264:refnum<queue>)  [unwired: 11 in]
        n136 = Current VI's Menubar() -> (w257:refnum<k9>)
        n137 = call-by-ref "Start Asynchronous Call"(reference=w268, error in=w267, "STOP Queue in"=w264, "This Application"=w259, 8:"error in (no error)"=w262, "tcp data event"=w256, "Caller menu reference"=w257, "Caller VI ref"=w258) -> (reference out=w251:refnum<vi>, error out=w254:errorcluster)  [unwired: 5 in, 1 out]
        n138 = Bundle By Name(cluster=w261, "SuperGUI.SuperGUI ref"=w251, "SuperGUI.STOP queue"=w264) -> (w260:T21)
        n139 = call <vilib>:"Add State(s) to Queue__jki_lib_state_machine.vi"("State(s) in (\"\")"=w270) -> ("States Out"=w269:string)  [unwired: 14 in]
      }
      frame "UI: Stop SuperGUI" {
        # "Stop Supergui Clone and wait until it exit properly"
        n140 = call <vilib>:"Add State(s) to Queue__jki_lib_state_machine.vi"("State(s) in (\"\")"=w278) -> ("States Out"=w277:string)  [unwired: 14 in]
        n141 = Unbundle By Name(w273) -> ("SuperGUI.SuperGUI ref"=w275:refnum<vi>, "SuperGUI.STOP queue"=w274:refnum<queue>)
        n142 = Release Queue(queue=w274, error in (no error)=w272) -> (error out=w276:errorcluster)  [unwired: 1 in, 2 out]
        n143 = call-by-ref "Wait On Asynchronous Call"(reference=w275, error in=w276) -> ("error out"=w271:errorcluster)  [unwired: 11 in, 2 out]
      }
      frame "UI: Cursor Set" {
        # "Argument"
        # "Set and Unset Cursor Busy.\n(Usage: \"UI: Cursor Set >> Busy|Idle\")"
        n144 = call <vilib>:"Add State(s) to Queue__jki_lib_state_machine.vi"("State(s) in (\"\")"=w284) -> ("States Out"=w283:string)  [unwired: 14 in]
        n145 = case shown="\"Idle\", Default" w279 {
          tunnel: w281 -> [w286 w288]
          tunnel: [w285 w287] -> w280
          frame "Idle", Default {
            n146 = call <vilib>:"Unset Busy.vi"("error in (no error)"=w286) -> ("error out"=w285:errorcluster)  [unwired: 10 in]
          }
          frame "Busy" {
            n147 = call <vilib>:"Set Busy.vi"("error in (no error)"=w288) -> ("error out"=w287:errorcluster)  [unwired: 9 in, 1 out]
          }
        }
      }
      frame "UI: Front Panel State" {
        # "Argument"
        # "Set Front Panel Open or Closed\n(Usage: \"UI: Front Panel State >> Open|Close\")"
        n148 = call <vilib>:"Add State(s) to Queue__jki_lib_state_machine.vi"("State(s) in (\"\")"=w295) -> ("States Out"=w294:string)  [unwired: 14 in]
        n149 = Unbundle By Name(w291) -> ("Core.Current VI Reference"=w290:refnum<vi>)
        n150 = case shown="\"Open\", Default" w289 {
          tunnel: w293 -> [w299 w312]
          tunnel: [w301 w313] -> w292
          tunnel: w290 -> [w300 w310]
          frame "Open", Default {
            n151 = property class="VI"(reference=w300, error in=w299) -> (reference out=w297:refnum<vi>, error out=w298:errorcluster, "Front Panel.Open"=w296:bool)
            n152 = case shown="False" w296 {
              tunnel: [w304 w307] -> w301
              tunnel: w298 -> [w303 w307]
              tunnel: w297 -> [w302 _]
              frame False {
                n153 = invoke class="VI" method="FP.Open"(reference=w302, error in=w303, "Activate"=TRUE, "State"=T20."Standard") -> (error out=w304:errorcluster)  [unwired: 1 in, 4 out]
              }
              frame True {
              }
            }
          }
          frame "Close" {
            n154 = property class="VI"(reference=w310, error in=w312) -> (reference out=w309:refnum<vi>, error out=w311:errorcluster, "Front Panel.Open"=w308:bool)
            n155 = case shown="True" w308 {
              tunnel: [w314 w317] -> w313
              tunnel: w311 -> [w314 w316]
              tunnel: w309 -> [_ w315]
              frame False {
              }
              frame True {
                n156 = invoke class="VI" method="FP.Close"(reference=w315, error in=w316) -> (error out=w317:errorcluster)  [unwired: 1 in, 2 out]
              }
            }
          }
        }
      }
      frame "---------- Macro ----------" {
        # "Do not put any code in this frame.\n(It is a separator no-op. You can make a copy of this frame to create a new Macro frame)"
        n157 = call <vilib>:"Add State(s) to Queue__jki_lib_state_machine.vi"("State(s) in (\"\")"=w321) -> ("States Out"=w320:string)  [unwired: 14 in]
      }
      frame "Macro: Initialize" {
        # "Initialization Macro\n(This is called once, when the VI starts)"
        n158 = call <vilib>:"Add State(s) to Queue__jki_lib_state_machine.vi"("State(s) in Front (\"\")"="Data: Initialize\nInitialize Core Data\nUI: Initialize\nUI: Get Device Name\nUI: Start SuperGUI\nUI: Front Panel State >> Open", "State(s) in (\"\")"=w326) -> ("States Out"=w325:string)  [unwired: 13 in]
      }
      frame "Macro: Exit" {
        # "Exit Macro\n(This is called once, when the VI exits)"
        n159 = Unbundle By Name(w334) -> ("Core.Close Panel on Exit?"=w333:bool)
        n160 = Select(t="UI: Front Panel State >> Close", s=w333, f="") -> (s? t:f=w330:string)
        n161 = call <vilib>:"Add State(s) to Queue__jki_lib_state_machine.vi"("State(s) in Front (\"\")"="UI: Stop SuperGUI" ("State(s) in Front (\"\")"), "State(s) in (\"\")"=w330, "State(s) at Back (\"\")"="Data: Cleanup\nExit") -> ("States Out"=w328:string)  [unwired: 12 in]
        n162 = call <vilib>:"Add State(s) to Queue__jki_lib_state_machine.vi"("State(s) in Front (\"\")"=w328, "State(s) in (\"\")"=w337) -> ("States Out"=w336:string)  [unwired: 13 in]
      }
      frame "---------- New Category ----------" {
        # "Template Separator\n(You can make a copy of, or modify, this frame)"
        n163 = call <vilib>:"Add State(s) to Queue__jki_lib_state_machine.vi"("State(s) in (\"\")"=w341) -> ("States Out"=w340:string)  [unwired: 14 in]
      }
      frame "New Category: 1" {
        # "Your code here.\n(You can make a copy of, or modify, this frame)"
        n164 = call <vilib>:"Add State(s) to Queue__jki_lib_state_machine.vi"("State(s) in (\"\")"=w345) -> ("States Out"=w344:string)  [unwired: 14 in]
      }
      frame "New Category: 2" {
        # "Your code here.\n(You can make a copy of, or modify, this frame)"
        n165 = call <vilib>:"Add State(s) to Queue__jki_lib_state_machine.vi"("State(s) in (\"\")"=w349) -> ("States Out"=w348:string)  [unwired: 14 in]
      }
    }
  }
